vi "VG-checkComPort.vi"(8 "error in (no error)":errorcluster, 10 "connection settings":T1={"Com"="", "baud rate (9600)"=38400} {"baud rate (9600)" items=["75"=75, "110"=110, "134"=134, "150"=150, "300"=300, "600"=600, "1200"=1200, "1800"=1800, "2400"=2400, "4800"=4800, "7200"=7200, "9600"=9600, "14400"=14400, "19200"=19200, "28800"=28800, "38400"=38400, "56000"=56000, "57600"=57600, "115200"=115200, "128000"=128000, "230400"=230400]}, 11 "VG-VNA_GUI in":refnum<class "VG-VNA_GUI.lvclass">) -> (0 "error out":errorcluster, 1 "Com Port Found?":bool, 2 "connection settings dup":T1={"Com"="", "baud rate (9600)"=38400} {"baud rate (9600)" items=["75"=75, "110"=110, "134"=134, "150"=150, "300"=300, "600"=600, "1200"=1200, "1800"=1800, "2400"=2400, "4800"=4800, "7200"=7200, "9600"=9600, "14400"=14400, "19200"=19200, "28800"=28800, "38400"=38400, "56000"=56000, "57600"=57600, "115200"=115200, "128000"=128000, "230400"=230400]}, 3 "VG-VNA_GUI out":refnum<class "VG-VNA_GUI.lvclass">)   [LabVIEW 2020, in "VG-VNA_GUI.lvlib" / "VG-VNA_GUI.lvclass"]
uses:
  VG-VNA_GUI.lvclass
  classes/vna-drivers/liteVNA/VD-connection_settings.ctl
  classes/hardware-protocol/serial/HP-S-baudrate.ctl
  classes/hardware-protocol/serial/HP-S-Serial.lvclass
  classes/vna-drivers/liteVNA/VD-LV-LiteVNA.lvclass
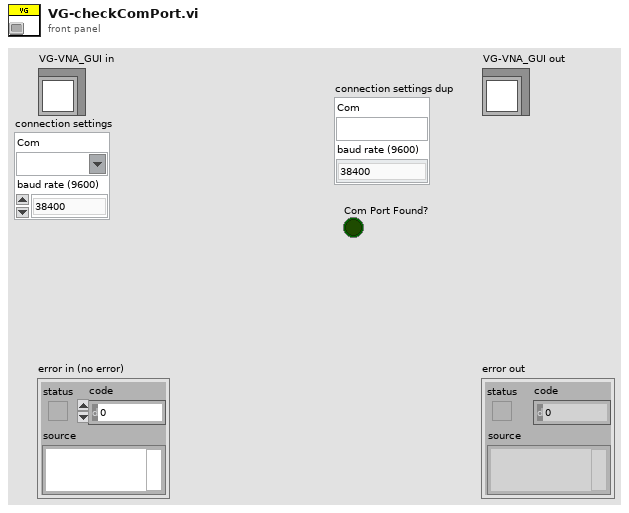
[diagram p1: front panel]
types:
  T1 = typedef "VD-LV-LiteVNA.lvclass/VD-connection_settings.ctl" = cluster{"Com":refnum<visa-resource-name>, "baud rate (9600)":T2}
  T2 = typedef "HP-S-Serial.lvclass/HP-S-baudrate.ctl" = u32
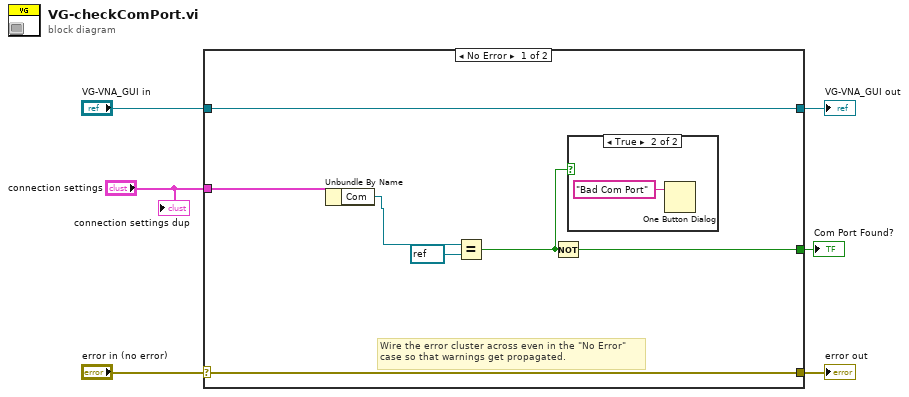
[diagram p0: block diagram]
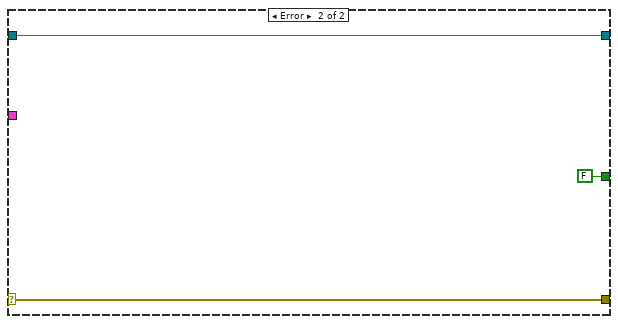
[diagram p3: hidden frame]
diagram:
  n1 = case shown="No Error" "error in (no error)" {
    selector: "error in (no error)" -> [w12 w17]
    tunnel: [w12 w17] -> w5
    tunnel: [w13 w16] -> w3
    tunnel: "VG-VNA_GUI in" -> [w13 w16]
    tunnel: "connection settings" -> [w11 _]
    tunnel: [w8 FALSE] -> w1
    frame No Error {
      # "Wire the error cluster across even in the \"No Error\"\ncase so that warnings get propagated."
      n2 = Unbundle By Name(w11) -> ("Com"=w10:refnum<visa-resource-name>)
      n3 = Equal?(x=w10, y=refnum<visa-resource-name> refnum) -> (x = y?=w7:bool)
      n4 = Not(x=w7) -> (.not. x?=w8:bool)
      n5 = case shown="True" w7 {
        frame False {
        }
        frame True {
          n6 = One Button Dialog(message="Bad Com Port") -> ()  [unwired: 1 in, 1 out]
        }
      }
    }
    frame Error {
    }
  }
  "error out" <- w5
  "VG-VNA_GUI out" <- w3
  "Com Port Found?" <- w1
  "connection settings dup" <- "connection settings"
